vi "Tracepoint_UnexpectedValue.vi"(4 "region bounds":string, 5 "camera":string, 6 "image stats":string, 7 "tracepoint id":string, 8 "error in (no error)":errorcluster, 9 "Value":dbl, 10 "Value":sgl, 11 "Qbus":refnum<class "Qbus.lvclass">) -> (0 "error out":errorcluster)   [LabVIEW 2017, in "IrAnalysis.lvlib"]
uses:
  <vilib>/addons/InsightCM/Devices/Shared/Ir/IrAnalysis/IrAnalysis.lvlib
  <vilib>/addons/Qbus/Qbus.lvclass
  <vilib>/addons/TraceLogger/TraceLogger.lvlib
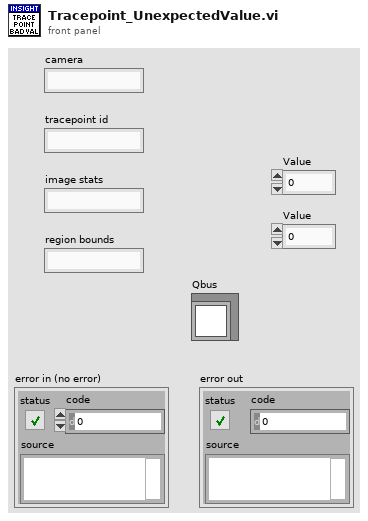
[diagram p1: front panel]
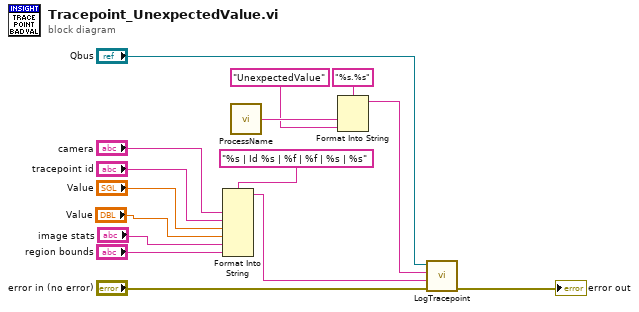
[diagram p0: block diagram]
diagram:
  n1 = Format Into String(format string="%s | Id %s | %f | %f | %s | %s", "camera", "tracepoint id", "Value", "Value", "image stats", "region bounds") -> (resulting string=w13:string)  [unwired: 2 in, 1 out]
  n2 = call <vilib>:"ProcessName.vi"() -> ("process name"=w11:string)  [unwired: 5 in]
  n3 = Format Into String(format string="%s.%s", w11, "UnexpectedValue" ("ProcessName")) -> (resulting string=w8:string)  [unwired: 2 in, 1 out]
  n4 = call <vilib>:"LogTracepoint.vi"("error in (no error)"="error in (no error)", "log string"=w13, "tracepoint"=w8, "qbus in"="Qbus") -> ("error out"=→"error out":errorcluster)  [unwired: 6 in, 1 out]
